vi "uarv2.vi"() -> ()   [LabVIEW 2023]
panel:
  out "Slucajan broj":dbl
  in  "Unesite broj":i32
  out "Array 2":i32[](array[numeric])
  out "Whole Array":i32[][](array[numeric])
  out "Array element":dbl
  out "appended array":dbl[][](array[numeric])
  out "Numeric":i32
  in  "Array":i32[][](array[numeric])
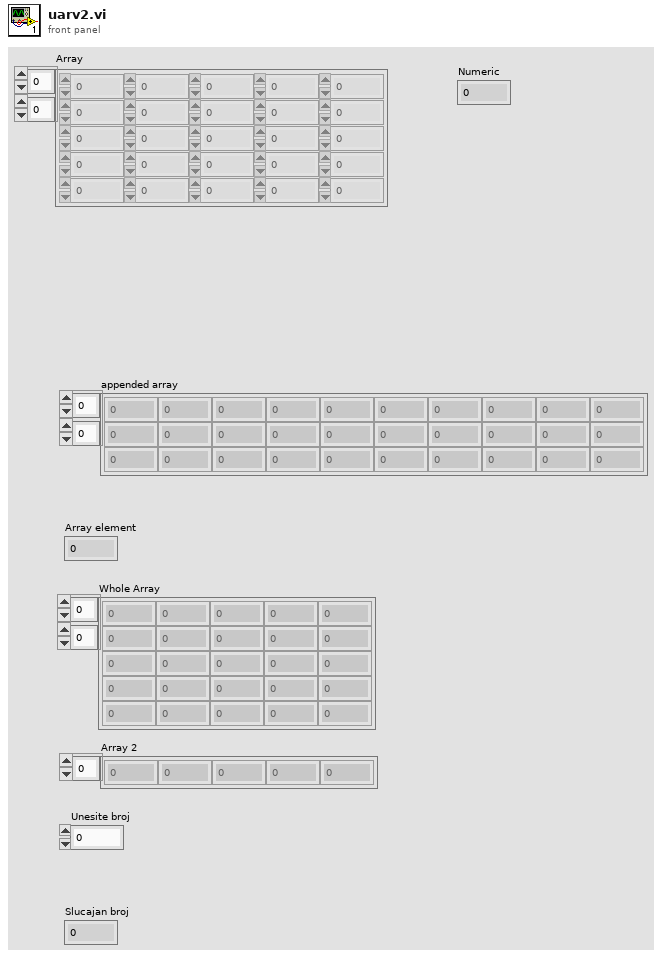
[diagram p1: front panel]
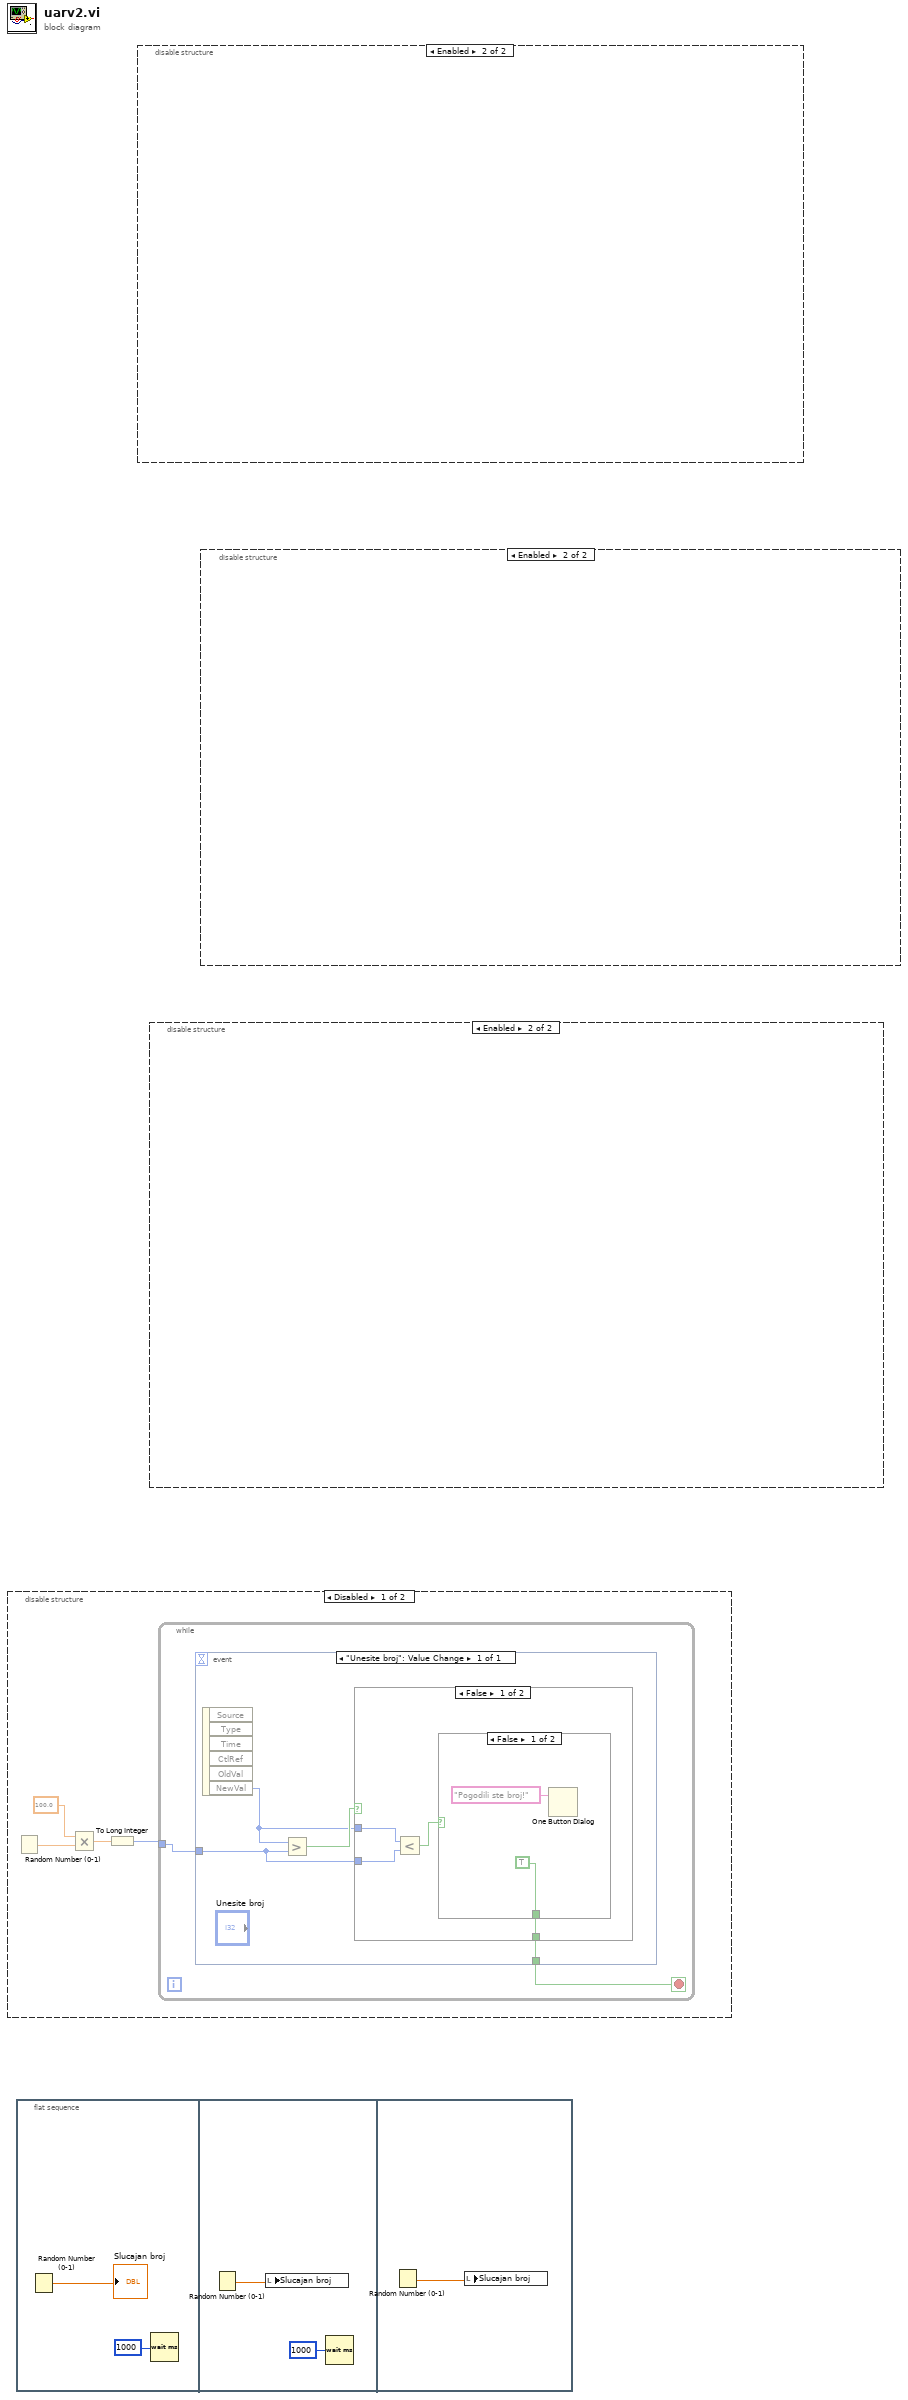
[diagram p0: block diagram]
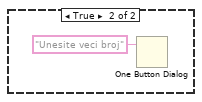
[diagram p2: hidden frame]
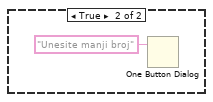
[diagram p3: hidden frame]
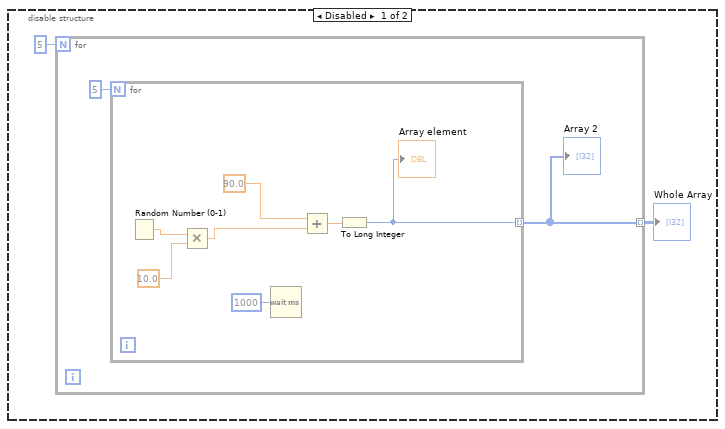
[diagram p5: hidden frame]
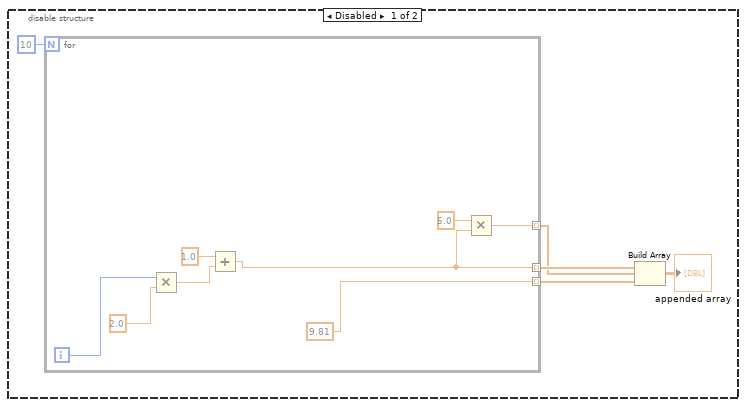
[diagram p6: hidden frame]
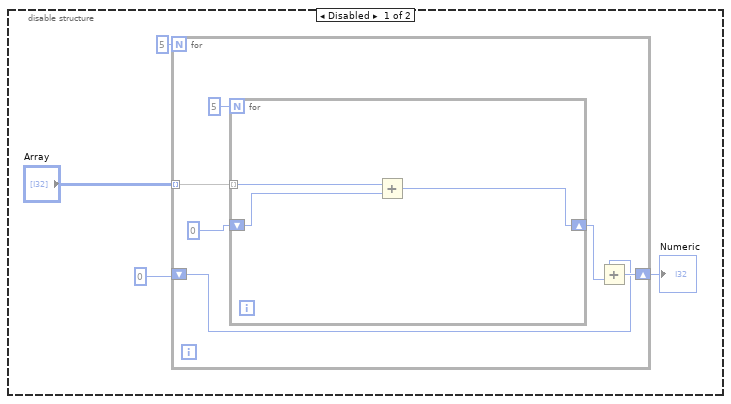
[diagram p7: hidden frame]
diagram:
  n1 = disable-structure shown="Disabled" {
    frame Disabled {
      n2 = Random Number (0-1)() -> (number: 0 to 1=w4:dbl)
      n3 = Multiply(x=100.0, y=w4) -> (x*y=w1:dbl)
      n4 = To Long Integer(number=w1) -> (32bit integer=w2:i32)
      n5 = while {
        tunnel: w2 -> [w6]
        stop <- w5 stop-if-true
        n6 = event shown="[0] \"Unesite broj\": Value Change" {
          selector: _ -> [_]
          dyn-events: _ -> [_]
          timeout: _ -> [_]
          tunnel: w6 -> [w9]
          tunnel: [w7] -> w5
          event "Unesite broj": Value Change {
            n7 = event-data() -> ("NewVal"=w8:i32)  [unwired: 1 in, 5 out]
            n8 = Greater?(x=w8, y=w9) -> (0:w10:bool)
            n9 = case shown="False" w10 {
              tunnel: w9 -> [w14 _]
              tunnel: w8 -> [w13 _]
              tunnel: [w11 _] -> w7
              frame False {
                n10 = Less?(x=w13, y=w14) -> (x < y?=w12:bool)
                n11 = case shown="False" w12 {
                  tunnel: [TRUE _] -> w11
                  frame False {
                    n12 = One Button Dialog(message="Pogodili ste broj!") -> ()  [unwired: 1 in, 1 out]
                  }
                  frame True {
                    n13 = One Button Dialog(message="Unesite veci broj") -> ()  [unwired: 1 in, 1 out]
                  }
                }
              }
              frame True {
                n14 = One Button Dialog(message="Unesite manji broj") -> ()  [unwired: 1 in, 1 out]
              }
            }
          }
        }
      }
    }
    frame Enabled {
    }
  }
  n15 = flat-sequence {
    frame #0 {
      n16 = Random Number (0-1)() -> (number: 0 to 1=→"Slucajan broj":dbl)
      n17 = Wait (ms)(milliseconds to wait=u32 1000) -> ()  [unwired: 1 out]
    }
    frame #1 {
      n18 = Random Number (0-1)() -> (number: 0 to 1=w22:dbl)
      n19 = local write "Slucajan broj"(w22) -> ()
      n20 = Wait (ms)(milliseconds to wait=u32 1000) -> ()  [unwired: 1 out]
    }
    frame #2 {
      n21 = Random Number (0-1)() -> (number: 0 to 1=w23:dbl)
      n22 = local write "Slucajan broj"(w23) -> ()
    }
  }
  n23 = disable-structure shown="Enabled" {
    frame Disabled {
      n24 = for {
        N: 5 -> [_]
        tunnel: "Array" -> [w32] mode=indexing
        shift-right: [w29] -> w24
        shift-left: 0 -> [w28]
        n25 = for {
          N: 5 -> [_]
          tunnel: w32 -> [w36] mode=indexing
          shift-right: [w34] -> w30
          shift-left: 0 -> [w35]
          n26 = Add(x=w36, y=w35) -> (x+y=w34:i32)
        }
        n27 = Add(x=w28, y=w30) -> (x+y=w29:i32)
      }
      "Numeric" <- w24
    }
    frame Enabled {
    }
  }
  n28 = disable-structure shown="Enabled" {
    frame Disabled {
      n29 = for {
        N: 5 -> [_]
        tunnel: [w39] -> w37 mode=indexing
        n30 = for {
          N: 5 -> [_]
          tunnel: [w44] -> w39 mode=indexing
          n31 = Random Number (0-1)() -> (number: 0 to 1=w42:dbl)
          n32 = Multiply(x=w42, y=10.0) -> (x*y=w43:dbl)
          n33 = Wait (ms)(milliseconds to wait=u32 1000) -> ()  [unwired: 1 out]
          n34 = Add(x=90.0, y=w43) -> (x+y=w46:dbl)
          n35 = To Long Integer(number=w46) -> (32bit integer=w44:i32)
          "Array element" <- w44
        }
        "Array 2" <- w39
      }
      "Whole Array" <- w37
    }
    frame Enabled {
    }
  }
  n36 = disable-structure shown="Enabled" {
    frame Disabled {
      n37 = for {
        N: 10 -> [_]
        tunnel: [w55] -> w51 mode=indexing
        tunnel: [9.81] -> w50 mode=indexing
        tunnel: [w53] -> w48 mode=indexing
        i -> [w59]
        n38 = Multiply(x=w59, y=2.0) -> (x*y=w58:dbl)
        n39 = Add(x=1.0, y=w58) -> (x+y=w55:dbl)
        n40 = Multiply(x=5.0, y=w55) -> (x*y=w53:dbl)
      }
      n41 = Build Array(w51, w48, w50) -> (→"appended array":dbl[][])
    }
    frame Enabled {
    }
  }
